vi "test-vi-1.vi"() -> ()   [LabVIEW 2016, in "test-find-vi-by-name.lvlib"]
uses:
  test-find-vi-by-name.lvlib
panel:
  in  "test-ctl":dbl
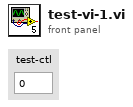
[diagram p1: front panel]
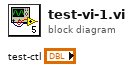
[diagram p0: block diagram]
diagram:
